vi "svm_add_problem_padding.vi"(8 "error in (no error)":errorcluster, 11 "problem":T1) -> (0 "error out":errorcluster, 3 "padded problem":T3)   [LabVIEW 2014]
uses:
  Controls/svm_problem_padded.ctl
  Controls/svm_node_padded.ctl
  Controls/svm_problem.ctl
  Controls/svm_node.ctl
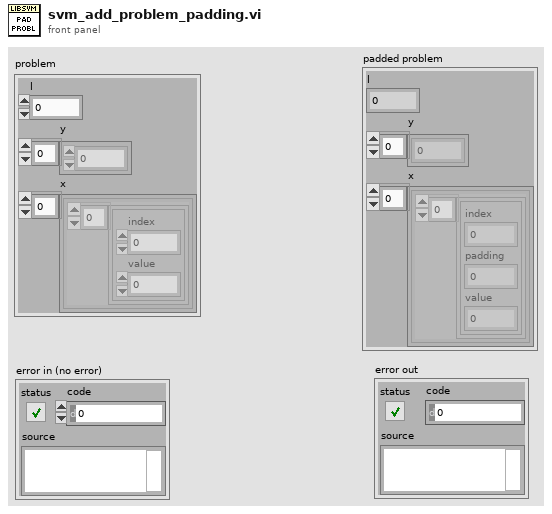
[diagram p1: front panel]
types:
  T1 = typedef "svm_problem.ctl" = cluster{"l":i32, "y":dbl[], "x":cluster{T2[]}[]}
  T2 = typedef "svm_node.ctl" = cluster{"index":i32, "value":dbl}
  T3 = typedef "svm_problem_padded.ctl" = cluster{"l":i32, "y":dbl[], "x":cluster{T4[]}[]}
  T4 = typedef "svm_node_padded.ctl" = cluster{"index":i32, "padding":i32, "value":dbl}
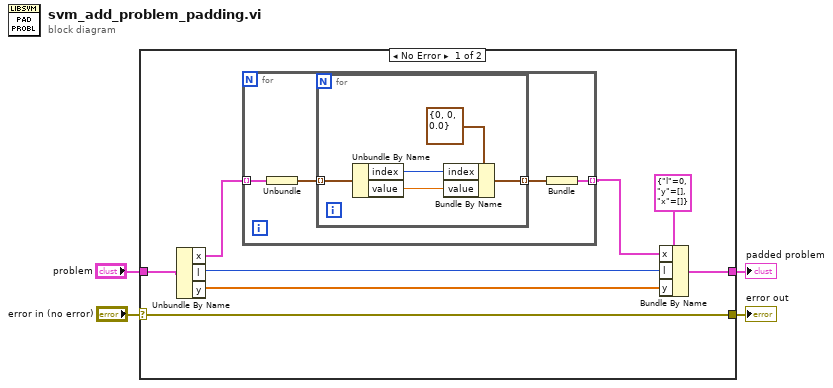
[diagram p0: block diagram]
diagram:
  n1 = case shown="No Error" "error in (no error)" {
    selector: "error in (no error)" -> [w8 w22]
    tunnel: [w8 w22] -> w3
    tunnel: [w6 _] -> w2
    tunnel: "problem" -> [w5 _]
    frame No Error {
      n2 = Unbundle By Name(w5) -> ("x"=w12:cluster{T2[]}[], "l"=w10:i32, "y"=w9:dbl[])
      n3 = for {
        tunnel: w12 -> [w16] mode=indexing
        tunnel: [w13] -> w11 mode=indexing
        n4 = Unbundle(w16) -> (w15:T2[])
        n5 = for {
          tunnel: w15 -> [w21] mode=indexing
          tunnel: [w18] -> w14 mode=indexing
          n6 = Unbundle By Name(w21) -> ("index"=w20:i32, "value"=w19:dbl)
          n7 = Bundle By Name(cluster=T4 {"index"=0, "padding"=0, "value"=0.0} ("svm_node"), "index"=w20, "value"=w19) -> (w18:T4)
        }
        n8 = Bundle(w14) -> (w13:cluster{T4[]})  [unwired: 1 in]
      }
      n9 = Bundle By Name(cluster=T3 {"l"=0, "y"=[], "x"=[]} ("svm_problem"), "x"=w11, "l"=w10, "y"=w9) -> (w6:T3)
    }
    frame Error {
    }
  }
  "error out" <- w3
  "padded problem" <- w2
